vi "test_color_plus_grand.vi"(8 "limite inférieure":dbl, 11 "signal":dbl(knob) scale=0.0..10.0) -> (0 "result color":u32)   [LabVIEW 2013]
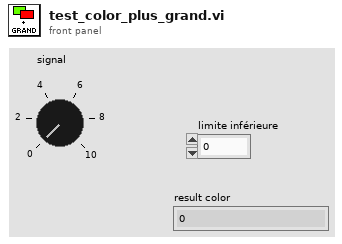
[diagram p1: front panel]
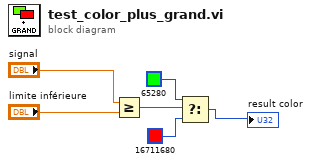
[diagram p0: block diagram]
diagram:
  n1 = Greater Or Equal?(x="signal", y="limite inférieure") -> (x >= y?=w6:bool)
  n2 = Select(t=u32 65280, s=w6, f=u32 16711680) -> (s? t:f=→"result color":u32)
